vi "Keithley2612b_IV_vg_vd_loop_indexing.vi"(3 "Error Query (False)":bool, 4 "Limit":dbl=1.0, 7 "Source Function (Current)":enum32{"Current", "Voltage"}(ring)=enum."Voltage", 8 "error in (no error)":errorcluster, 9 "Channel (Channel A)":T1, 10 "Node (0-64)":i8 min=0 max=64 step=1, 11 "VISA resource name":refnum<visa-resource-name>) -> (0 "error out":errorcluster)   [LabVIEW 2016]
doc: "This example shows how to configure the source and take a measurement."
uses:
  <instrlib>/Keithley 2600 Series/Public/Channel.ctl
  <vilib>/express/express shared/transition.llb/Dynamic To Waveform Array.vi
  <vilib>/express/express signal manip/GetorSetDDTAttributes/Set DDT Attributes/SetT0.vi
  <vilib>/express/express shared/transition.llb/Waveform Array To Dynamic.vi
  <vilib>/express/express signal manip/GetorSetDDTAttributes/Set DDT Attributes/Set DDT Properties.xnode
  <instrlib>/Keithley 2600 Series/Keithley 2600 Series.lvlib
panel:
  in  "Delay (s) 2":dbl
  in  "Step Size 2":dbl
  in  "End Voltage 2":dbl
  in  "Start Voltage 2":dbl
  in  "Limit 2":dbl=1.0
  out "Current Output 2":string
  out "Voltage Output 2":string
  out "Current Number Past 2":dbl
  in  "Source Function (Current) 2":enum32{"Current", "Voltage"}(ring)=enum."Voltage"
  in  "Channel (Channel A) 2":T1
  out "Current Number Past":dbl
  out "Voltage Output":string
  out "Current Output":string
  in  "Delay (s)":dbl
  in  "Step Size":dbl
  in  "End Voltage":dbl
  in  "Start Voltage":dbl
  # "(c) 2008 Keithley Instruments, Inc.  ALL RIGHTS RESERVED."
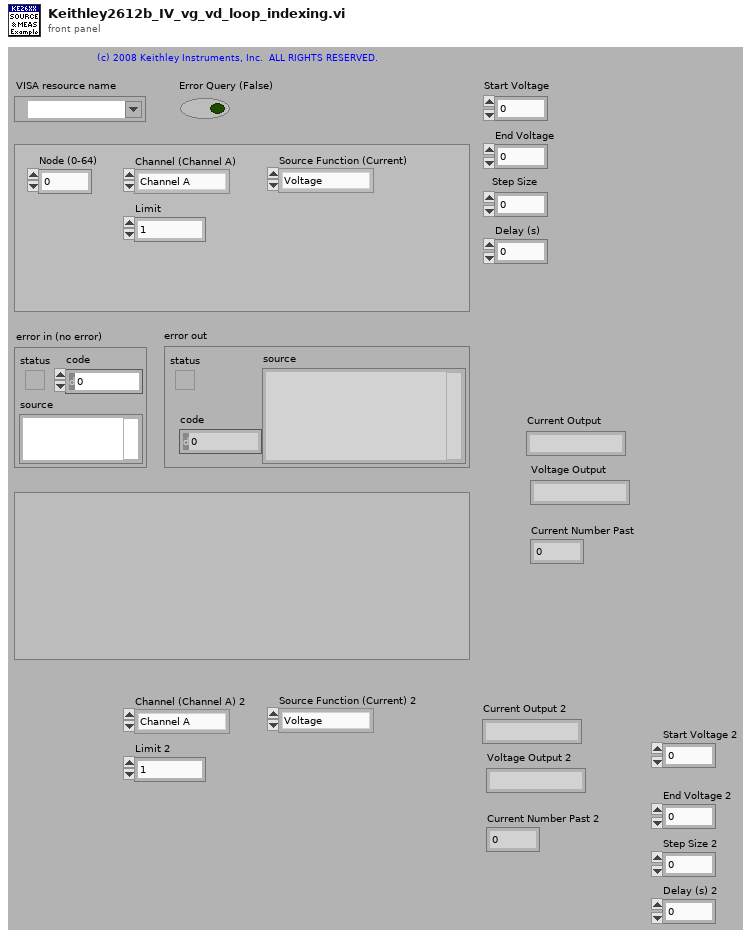
[diagram p1: front panel]
types:
  T1 = typedef "Keithley 2600 Series.lvlib/Channel.ctl" = enum32{"Channel A", "Channel B"}
  T2 = typedef "NI_Matrix.lvlib/RealMatrix.ctl" = dbl[][]
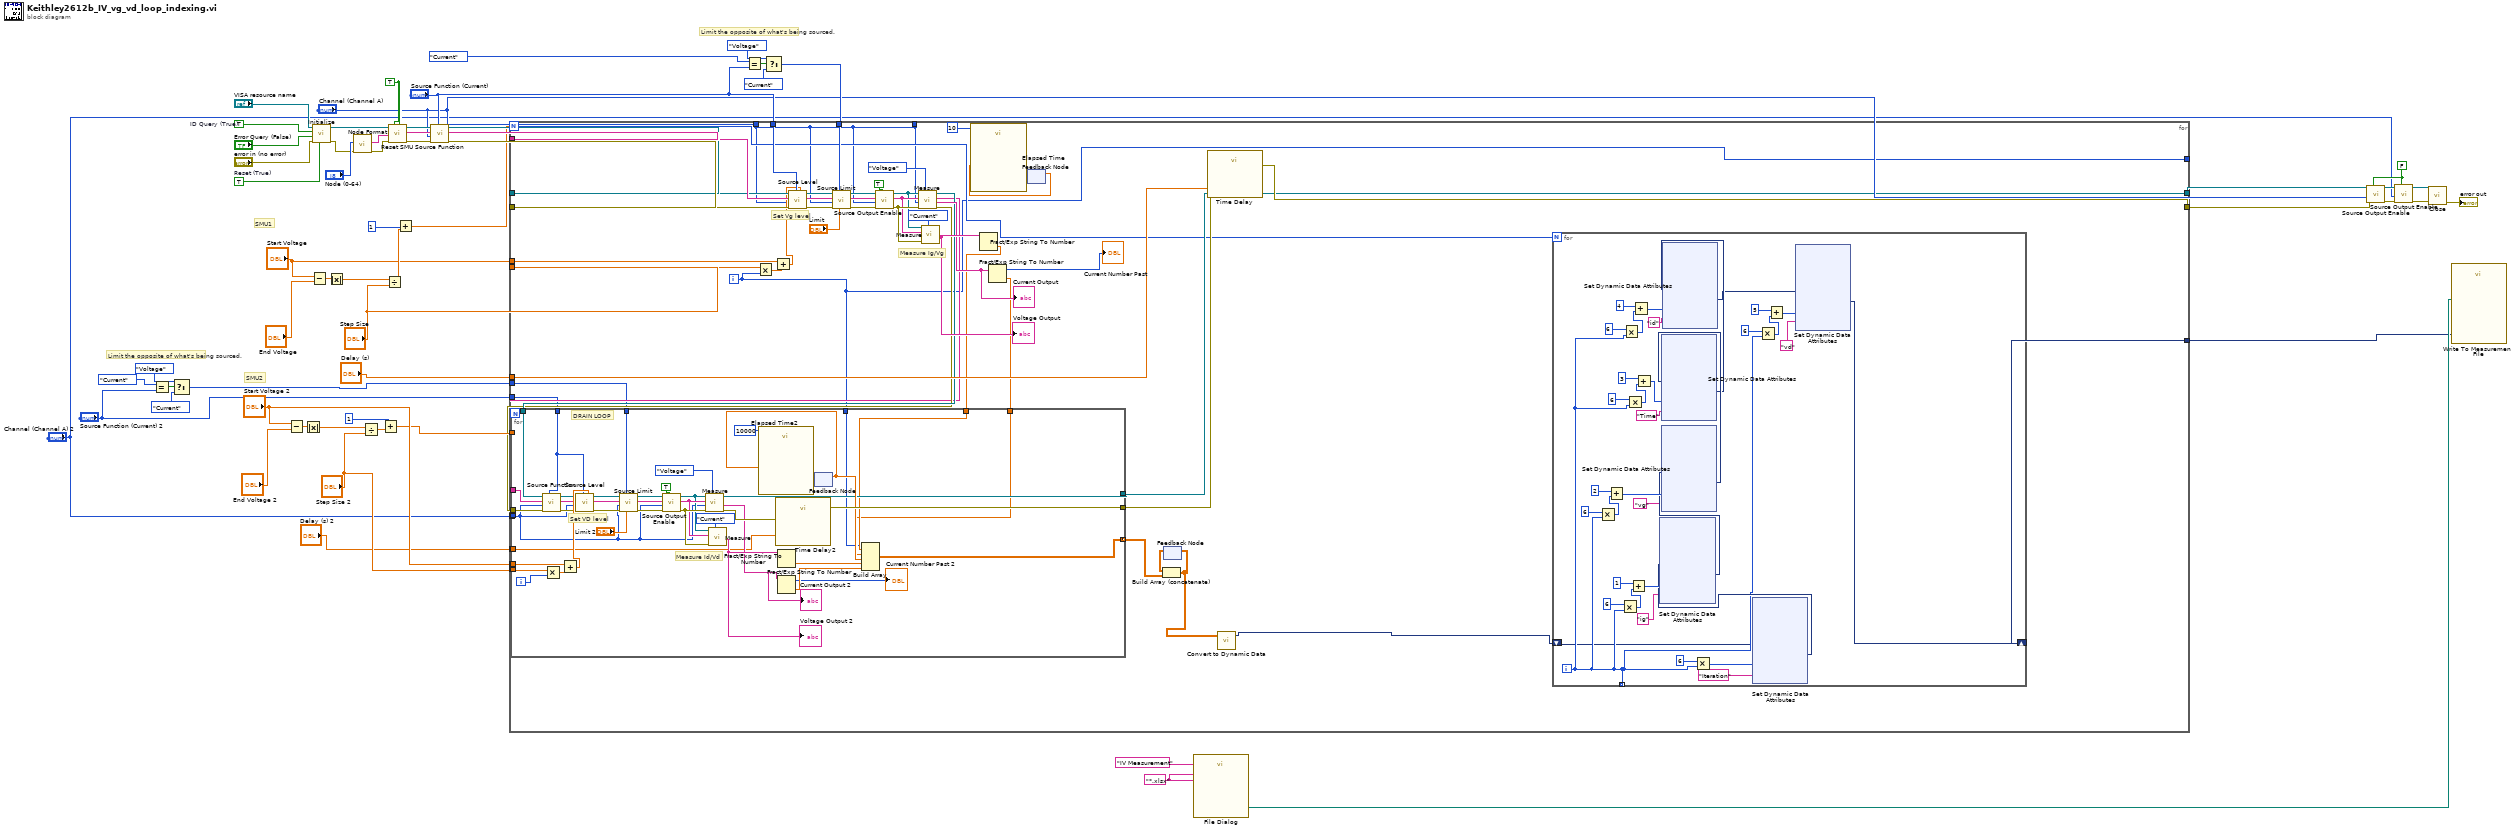
[diagram p0: block diagram]
diagram:
  w13 = "*.xlsx"
  w27 = TRUE
  w6 = FALSE ("Output (Off)")
  w58 = TRUE  # Reset (True)
  w61 = TRUE  # ID Query (True)
  # "SMU2"
  # "SMU1"
  # "Limit the opposite of what's being sourced."
  # "Limit the opposite of what's being sourced."
  n1 = Equal?(x=enum32{"Current", "Voltage"}."Current", y="Source Function (Current) 2") -> (x = y?=w33:bool)
  n2 = Select(t=enum32{"Current", "Voltage"}."Voltage" ("x"), s=w33, f=enum32{"Current", "Voltage"}."Current") -> (s? t:f=w14:enum32{"Current", "Voltage"})
  n3 = Subtract(x="Start Voltage 2", y="End Voltage 2") -> (x-y=w22:dbl)
  n4 = Absolute Value(x=w22) -> (abs(x)=w21:dbl)
  n5 = Subtract(x="Start Voltage", y="End Voltage") -> (x-y=w41:dbl)
  n6 = call <instrlib>:"Initialize.vi"("Reset (True)"=w58, "error in (no error)"="error in (no error)", "Error Query (False)"="Error Query (False)", "ID Query (True)"=w61, "VISA resource name"="VISA resource name") -> ("error out"=w35:errorcluster, "VISA resource name out"=w28:refnum<visa-resource-name>)  [unwired: 1 in, 4 out]
  n7 = Absolute Value(x=w41) -> (abs(x)=w40:dbl)
  n8 = call <instrlib>:"Node Format.vi"("error in"=w35, "Node (0-64)"="Node (0-64)") -> ("error out"=w54:errorcluster, "Formatted Node"=w55:string)  [unwired: 8 out]
  n9 = Divide(x=w21, y="Step Size 2") -> (x/y=w19:dbl)
  n10 = Add(x=1, y=w19) -> (x+y=w11:dbl)
  n11 = Divide(x=w40, y="Step Size") -> (x/y=w38:dbl)
  n12 = call <instrlib>:"Reset SMU.vi"("SMU B (No)"=w27, "SMU A (No)"=w27, "error in (no error)"=w54, "Node In"=w55, "VISA resource name"=w28) -> ("error out"=w26:errorcluster, "Node Out"=w24:string, "VISA resource name out"=w25:refnum<visa-resource-name>)  [unwired: 4 out]
  n13 = Add(x=1, y=w38) -> (x+y=w1:dbl)
  n14 = call <instrlib>:"Source Function.vi"("Function (Current)"="Source Function (Current)", "error in (no error)"=w26, "Channel (Channel A)"="Channel (Channel A)", "Node In"=w24, "VISA resource name"=w25) -> ("error out"=w52:errorcluster, "Node Out"=w51:string, "VISA resource name out"=w50:refnum<visa-resource-name>)  [unwired: 4 out]
  n15 = Equal?(x=enum32{"Current", "Voltage"}."Current", y="Source Function (Current)") -> (x = y?=w56:bool)
  n16 = Select(t=enum32{"Current", "Voltage"}."Voltage" ("x"), s=w56, f=enum32{"Current", "Voltage"}."Current") -> (s? t:f=w44:enum32{"Current", "Voltage"})
  n17 = for {
    N: w1 -> [w65]
    tunnel: w52 -> [w105]
    tunnel: w51 -> [w104]
    tunnel: w50 -> [w103]
    tunnel: "Channel (Channel A)" -> [w62]
    tunnel: "Source Function (Current)" -> [w100]
    tunnel: "Step Size" -> [w96]
    tunnel: "Start Voltage" -> [w101]
    tunnel: w44 -> [w99]
    tunnel: [w76] -> w9
    tunnel: [w97] -> w8
    tunnel: "Delay (s)" -> [w98]
    tunnel: "Step Size 2" -> [w80]
    tunnel: "Start Voltage 2" -> [w79]
    tunnel: w11 -> [w78]
    tunnel: "Delay (s) 2" -> [w75]
    tunnel: "Channel (Channel A) 2" -> [w74]
    tunnel: "Source Function (Current) 2" -> [w73]
    tunnel: w14 -> [w72]
    tunnel: [w66] -> w2
    tunnel: [w63] -> _
    tunnel: [w62] -> _
    i -> [w63]
    # "Measure Ig/Vg"
    # "Set Vg level"
    n18 = Multiply(x=w96, y=w63) -> (x*y=w102:dbl)
    n19 = Add(x=w101, y=w102) -> (x+y=w84:dbl)
    n20 = call <instrlib>:"Source Level.vi"("Level (0.000)"=w84, "Function (Current)"=w100, "error in (no error)"=w105, "Channel (Channel A)"=w62, "Node In"=w104, "VISA resource name"=w103) -> ("error out"=w106:errorcluster, "Node Out"=w111:string, "VISA resource name out"=w107:refnum<visa-resource-name>)  [unwired: 3 out]
    n21 = call <instrlib>:"Source Limit.vi"("Limit (0.000)"="Limit", "Function (Current)"=w99, "error in (no error)"=w106, "Channel (Channel A)"=w62, "Node In"=w111, "VISA resource name"=w107) -> ("error out"=w109:errorcluster, "Node Out"=w112:string, "VISA resource name out"=w108:refnum<visa-resource-name>)  [unwired: 3 out]
    n22 = call <instrlib>:"Source Output Enable.vi"("Output (Off)"=TRUE, "error in (no error)"=w109, "Channel (Channel A)"=w62, "Node In"=w112, "VISA resource name"=w108) -> ("error out"=w94:errorcluster, "Node Out"=w93:string, "VISA resource name out"=w92:refnum<visa-resource-name>)  [unwired: 4 out]
    n23 = call <instrlib>:"Measure.vi"("Function (Current)"=enum32{"Current", "Voltage"}."Voltage" ("x"), "error in (no error)"=w94, "Channel (Channel A)"=w62, "Node In"=w93, "VISA resource name"=w92) -> ("error out"=w82:errorcluster, "Output"=w88:string, "Node Out"=w81:string, "VISA resource name out"=w83:refnum<visa-resource-name>)  [unwired: 2 in, 1 out]
    "Current Output" <- w88
    n24 = call <instrlib>:"Measure.vi"("Function (Current)"=enum32{"Current", "Voltage"}."Current" ("x"), "error in (no error)"=w94, "Node In"=w93, "VISA resource name"=w92) -> ("Output"=w89:string)  [unwired: 3 in, 4 out]
    "Voltage Output" <- w89
    n25 = Fract/Exp String To Number(string=w89) -> (number=w71:dbl)  [unwired: 3 in, 1 out]
    n26 = Fract/Exp String To Number(string=w88) -> (offset past number=→"Current Number Past":i32, number=w70:dbl)  [unwired: 3 in]
    n27 = for {
      N: w78 -> [_]
      tunnel: w81 -> [w238]
      tunnel: w80 -> [w257]
      tunnel: w79 -> [w261]
      tunnel: w72 -> [w260]
      tunnel: [w242] -> w76
      tunnel: [w258] -> w77
      tunnel: w82 -> [w239]
      tunnel: w83 -> [w237]
      tunnel: w75 -> [w241]
      tunnel: w74 -> [w234]
      tunnel: w73 -> [w231]
      tunnel: w71 -> [w233]
      tunnel: w70 -> [w232]
      tunnel: [w229] -> w68 mode=concatenating
      tunnel: w63 -> [w228]
      i -> [w230]
      # "Set VD level"
      # "Measure Id/Vd"
      # "DRAIN LOOP"
      n28 = call <instrlib>:"Source Function.vi"("Function (Current)"=w231, "error in (no error)"=w239, "Channel (Channel A)"=w234, "Node In"=w238, "VISA resource name"=w237) -> ("error out"=w240:errorcluster, "Node Out"=w236:string, "VISA resource name out"=w235:refnum<visa-resource-name>)  [unwired: 4 out]
      n29 = Multiply(x=w257, y=w230) -> (x*y=w262:dbl)
      n30 = Add(x=w261, y=w262) -> (x+y=w243:dbl)
      n31 = call <instrlib>:"Source Level.vi"("Level (0.000)"=w243, "Function (Current)"=w231, "error in (no error)"=w240, "Channel (Channel A)"=w234, "Node In"=w236, "VISA resource name"=w235) -> ("error out"=w263:errorcluster, "Node Out"=w268:string, "VISA resource name out"=w264:refnum<visa-resource-name>)  [unwired: 3 out]
      n32 = call <instrlib>:"Source Limit.vi"("Limit (0.000)"="Limit 2", "Function (Current)"=w260, "error in (no error)"=w263, "Channel (Channel A)"=w234, "Node In"=w268, "VISA resource name"=w264) -> ("error out"=w266:errorcluster, "Node Out"=w269:string, "VISA resource name out"=w265:refnum<visa-resource-name>)  [unwired: 3 out]
      n33 = call <instrlib>:"Source Output Enable.vi"("Output (Off)"=TRUE, "error in (no error)"=w266, "Channel (Channel A)"=w234, "Node In"=w269, "VISA resource name"=w265) -> ("error out"=w255:errorcluster, "Node Out"=w254:string, "VISA resource name out"=w253:refnum<visa-resource-name>)  [unwired: 4 out]
      n34 = call <instrlib>:"Measure.vi"("Function (Current)"=enum32{"Current", "Voltage"}."Voltage" ("x"), "error in (no error)"=w255, "Channel (Channel A)"=w234, "Node In"=w254, "VISA resource name"=w253) -> ("error out"=w259:errorcluster, "Output"=w248:string, "VISA resource name out"=w242:refnum<visa-resource-name>)  [unwired: 2 in, 2 out]
      "Current Output 2" <- w248
      n35 = call <instrlib>:"Measure.vi"("Function (Current)"=enum32{"Current", "Voltage"}."Current" ("x"), "error in (no error)"=w255, "Node In"=w254, "VISA resource name"=w253) -> ("Output"=w250:string)  [unwired: 3 in, 4 out]
      "Voltage Output 2" <- w250
      n36 = call "Time Delay2"("error in (no error)"=w259, "Delay Time (s)"=w241) -> ("error out"=w258:errorcluster)  [unwired: 9 in]
      n37 = Fract/Exp String To Number(string=w248) -> (offset past number=→"Current Number Past 2":i32, number=w247:dbl)  [unwired: 3 in]
      n38 = Fract/Exp String To Number(string=w250) -> (number=w249:dbl)  [unwired: 3 in, 1 out]
      n39 = feedback #1() -> (w244:dbl)  [unwired: 1 in]
      n40 = call "Elapsed Time2"("Time Target (s)"=10000, "Set Start Time (s)"=w244) -> ("Elapsed Time (s)"=w251:dbl)  [unwired: 10 in, 7 out]
      n41 = feedback-in #1(w251) -> ()
      n42 = Build Array(w228, w233, w232, w244, w249, w247) -> (w229:T2)
    }
    n43 = feedback #2() -> (w85:dbl)  [unwired: 1 in]
    n44 = call "Elapsed Time"("Time Target (s)"=10, "Set Start Time (s)"=w85) -> ("Elapsed Time (s)"=w90:dbl)  [unwired: 10 in, 7 out]
    n45 = feedback-in #2(w90) -> ()
    n46 = feedback #3() -> (w69:T2)  [unwired: 1 in]
    n47 = Build Array (concatenate)(w69, w68) -> (w67:T2)
    n48 = feedback-in #3(w67) -> ()
    n49 = call "Time Delay"("error in (no error)"=w77, "Delay Time (s)"=w98) -> ("error out"=w97:errorcluster)  [unwired: 9 in]
    n50 = call "Convert to Dynamic Data"("2D Array"=w67) -> ("Dynamic Data Type"=w64:dynamicdata)  [unwired: 3 in]
    n51 = for {
      N: w65 -> [_]
      shift-right: [w116] -> w66
      shift-left: w64 -> [w114]
      tunnel: [w115] -> _ mode=indexing
      i -> [w115]
      n52 = Multiply(x=6, y=w115) -> (x*y=w142:i32)
      n53 = Add(x=2, y=w142) -> (x+y=w135:i32)
      n54 = Multiply(x=6, y=w115) -> (x*y=w145:i32)
      n55 = Multiply(x=6, y=w115) -> (x*y=w136:i32)
      n56 = Multiply(x=6, y=w115) -> (x*y=w139:i32)
      n57 = Add(x=1, y=w145) -> (x+y=w131:i32)
      n58 = Add(x=4, y=w136) -> (x+y=w130:i32)
      n59 = Add(x=3, y=w139) -> (x+y=w117:i32)
      n60 = Multiply(x=6, y=w115) -> (x*y=w148:i32)
      n61 = xnode "Set Dynamic Data Attributes"("Signals In"=w114, "Signal Index"=w148, "Signal Name"="Iteration") -> ("Signals Out"=w128:dynamicdata)  [unwired: 1 in, 1 out]
      n62 = xnode "Set Dynamic Data Attributes"("Signals In"=w128, "Signal Index"=w131, "Signal Name"="ig") -> ("Signals Out"=w127:dynamicdata)  [unwired: 1 in, 1 out]
      n63 = xnode "Set Dynamic Data Attributes"("Signals In"=w127, "Signal Index"=w135, "Signal Name"="vg") -> ("Signals Out"=w126:dynamicdata)  [unwired: 1 in, 1 out]
      n64 = xnode "Set Dynamic Data Attributes"("Signals In"=w126, "Signal Index"=w117, "Signal Name"="Time") -> ("Signals Out"=w125:dynamicdata)  [unwired: 1 in, 1 out]
      n65 = xnode "Set Dynamic Data Attributes"("Signals In"=w125, "Signal Index"=w130, "Signal Name"="id") -> ("Signals Out"=w124:dynamicdata)  [unwired: 1 in, 1 out]
      n66 = Multiply(x=6, y=w115) -> (x*y=w132:i32)
      n67 = Add(x=5, y=w132) -> (x+y=w129:i32)
      n68 = xnode "Set Dynamic Data Attributes"("Signals In"=w124, "Signal Index"=w129, "Signal Name"="vd") -> ("Signals Out"=w116:dynamicdata)  [unwired: 1 in, 1 out]
    }
  }
  n69 = call "File Dialog"("default name"="IV Measurement", "pattern (all files)"=w13, "pattern label"=w13) -> ("selected path"=w3:path)  [unwired: 9 in, 3 out]
  n70 = call <instrlib>:"Source Output Enable.vi"("Output (Off)"=w6, "error in (no error)"=w8, "Channel (Channel A)"="Channel (Channel A)", "VISA resource name"=w9) -> ("error out"=w7:errorcluster, "VISA resource name out"=w10:refnum<visa-resource-name>)  [unwired: 1 in, 5 out]
  n71 = call <instrlib>:"Source Output Enable.vi"("Output (Off)"=w6, "error in (no error)"=w7, "Channel (Channel A)"="Channel (Channel A) 2", "VISA resource name"=w10) -> ("error out"=w45:errorcluster, "VISA resource name out"=w46:refnum<visa-resource-name>)  [unwired: 1 in, 5 out]
  n72 = call <instrlib>:"Close.vi"("error in (no error)"=w45, "VISA resource name"=w46) -> ("error out"=→"error out":errorcluster)  [unwired: 9 out]
  n73 = call "Write To Measurement File"("Signals"=w2, "Filename"=w3) -> ()  [unwired: 15 in, 3 out]
